vi "Remove_Destination.vi"(6 "defaultDir in":string, 7 "dest tag":string, 8 "error in (no error)":errorcluster, 9 "source in":refnum<class "IB_Source.lvclass">[](array[class]), 10 "destinations in":refnum<class "IB_Destination.lvclass">[](array[class]), 11 "IB_DestTree in":refnum<class "IB_Tree_Dest.lvclass">) -> (0 "error out":errorcluster, 1 "source out":refnum<class "IB_Source.lvclass">[](array[class]), 2 "destinations out":refnum<class "IB_Destination.lvclass">[](array[class]), 3 "IB_DestTree out":refnum<class "IB_Tree_Dest.lvclass">, 4 "defaultDir out":string, 5 "edit":T1)   [LabVIEW 2020, in "IB_Tree_Dest.lvclass"]
uses:
  <vilib>/AppBuilder/IB_Classes/Tree_Dest/IB_Tree_Dest.lvclass
  <vilib>/AppBuilder/IB_Classes/Tree_Dest/IB_Tree_Dest.lvclass/IB_Tree_Dest.ctl
  <vilib>/AppBuilder/IB_Classes/Tree/IB_Tree.lvclass
  <vilib>/AppBuilder/IB_Classes/Destination/IB_Destination.lvclass
  <vilib>/AppBuilder/IB_Classes/Source/IB_Source.lvclass
  <vilib>/AppBuilder/IB_Classes/Tree_Dest/destEdits_operation.ctl
  <vilib>/AppBuilder/IB_Classes/Tree_Dest/destEdits_edit.ctl
  <vilib>/AppBuilder/IB_Classes/Tree_Dest/destEdits_remove.ctl
  e:/builds/penguin/labview/branches/2020/dev/dist/vi.lib/AppBuilder/IB_Classes/Tree/IB_Tree.lvclass
  e:/builds/penguin/labview/branches/2020/dev/dist/vi.lib/AppBuilder/IB_Classes/Tree_Dest/IB_Tree_Dest.lvclass
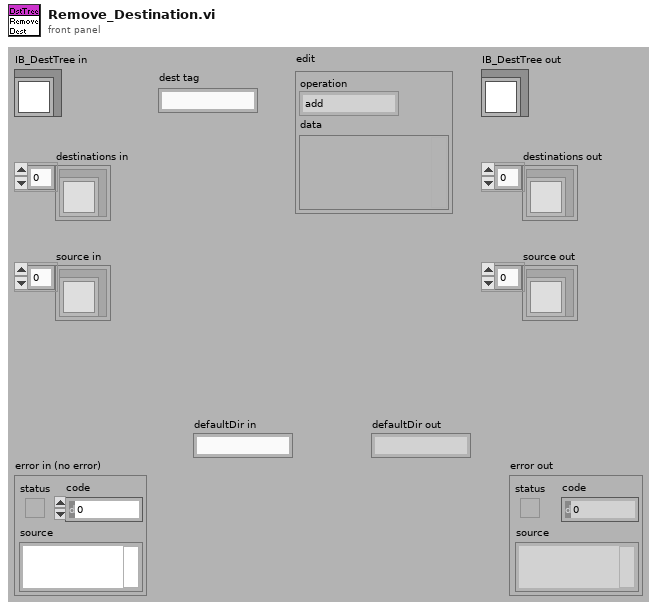
[diagram p1: front panel]
types:
  T1 = typedef "destEdits_edit.ctl" = cluster{"operation":T2, "data":variant}
  T2 = typedef "destEdits_operation.ctl" = enum16{"add", "remove", "rename", "sort children", "default dir changed"}
  T3 = typedef "destEdits_remove.ctl" = cluster{"child tag":string}
  T4 = typedef "IB_Source.ctl" = cluster{"name":string, "sourceTag":string, "destTag":string, "path":path, "eng_installPath":string, "UI_inBuild?":bool, "str ref?":bool}
  T5 = typedef "IB_Destination.ctl" = cluster{"name":string, "unlock":bool, "parentTag":string, "destTag":string, "eng_installPath":string}
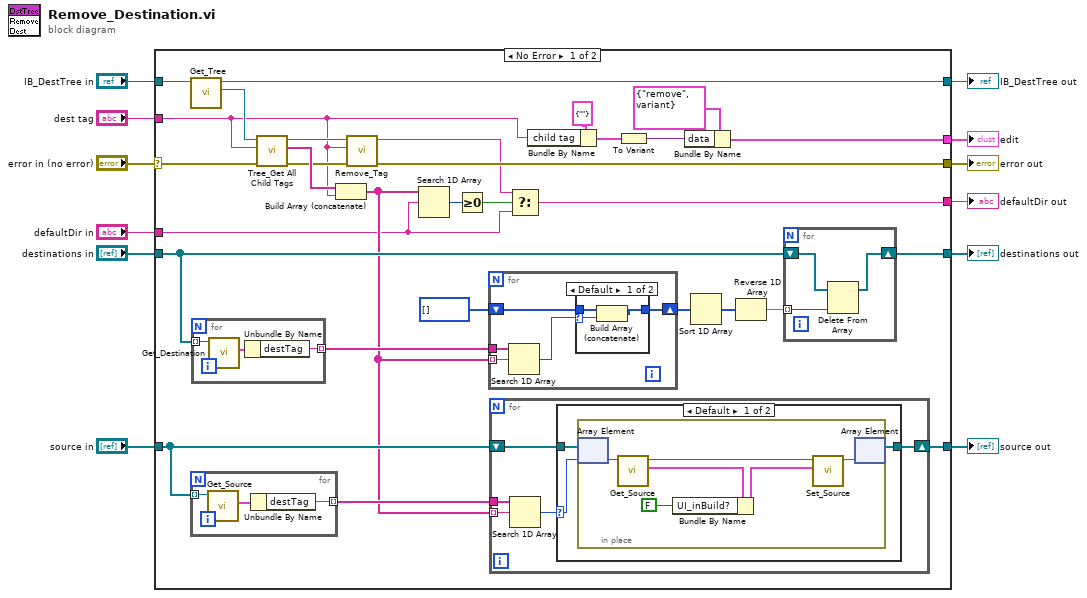
[diagram p0: block diagram]
diagram:
  n1 = case shown="No Error" "error in (no error)" {
    selector: "error in (no error)" -> [w38 w79]
    tunnel: [w29 w79] -> w11
    tunnel: [w40 w78] -> w9
    tunnel: "IB_DestTree in" -> [w41 w78]
    tunnel: "destinations in" -> [w33 w77]
    tunnel: "dest tag" -> [w18 _]
    tunnel: [w22 _] -> w6
    tunnel: [w32 w77] -> w5
    tunnel: "source in" -> [w21 w76]
    tunnel: [w20 w76] -> w3
    tunnel: "defaultDir in" -> [w15 _]
    tunnel: [w17 _] -> w1
    frame No Error {
      n2 = call <vilib>:"Get_Tree.vi"("IB_Tree in"=w41) -> ("ctl"=w42:refnum<vi>, "IB_Tree out"=w40:refnum<class "IB_Tree_Dest.lvclass">)  [unwired: 8 in, 1 out]
      n3 = for {
        tunnel: w21 -> [w60] mode=indexing
        tunnel: [w58] -> w30 mode=indexing
        n4 = call <vilib>:"Get_Source.vi"("IB_Source in"=w60) -> ("data"=w59:T4)  [unwired: 8 in, 2 out]
        n5 = Unbundle By Name(w59) -> ("destTag"=w58:string)
      }
      n6 = for {
        tunnel: w33 -> [w75] mode=indexing
        tunnel: [w73] -> w37 mode=indexing
        n7 = call <vilib>:"Get_Destination.vi"("IB_Destination in"=w75) -> ("data"=w74:T5)  [unwired: 8 in, 2 out]
        n8 = Unbundle By Name(w74) -> ("destTag"=w73:string)
      }
      n9 = call <vilib>:"Tree_Get All Child Tags.vi"("error in (no error)"=w38, "Parent Tag"=w18, "Tree Refnum"=w42) -> ("error out"=w28:errorcluster, "All Child Tags"=w39:string[], "dup Tree Refnum"=w27:refnum<vi>)  [unwired: 6 in]
      n10 = Build Array (concatenate)(w39, w18) -> (w16:string[])
      n11 = call <vilib>:"Remove_Tag.vi"("error in"=w28, "tag"=w18, "Tree Refnum"=w27) -> ("error out"=w29:errorcluster, "selected tag"=w19:string)  [unwired: 7 in]
      n12 = Search 1D Array(1D array=w16, element=w15) -> (index of element=w14:i32)  [unwired: 1 in]
      n13 = Greater Or Equal To 0?(x=w14) -> (x >= 0?=w13:bool)
      n14 = for {
        tunnel: w16 -> [w67] mode=indexing
        tunnel: w37 -> [w68]
        shift-right: [w64] -> w35
        shift-left: i32[] [] -> [w65]
        n15 = Search 1D Array(1D array=w68, element=w67) -> (index of element=w66:i32)  [unwired: 1 in]
        n16 = case shown="Default" w66 {
          selector: w66 -> [w69 _]
          tunnel: w65 -> [w71 w72]
          tunnel: [w70 w72] -> w64
          frame Default {
            n17 = Build Array (concatenate)(w71, w69) -> (w70:i32[])
          }
          frame -1 {
          }
        }
      }
      n18 = for {
        tunnel: w16 -> [w46] mode=indexing
        tunnel: w30 -> [w47]
        shift-right: [w43] -> w20
        shift-left: w21 -> [w44]
        n19 = Search 1D Array(1D array=w47, element=w46) -> (index of element=w45:i32)  [unwired: 1 in]
        n20 = case shown="Default" w45 {
          selector: w45 -> [w49 _]
          tunnel: w44 -> [w50 w57]
          tunnel: [w48 w57] -> w43
          frame Default {
            n21 = in-place {
              n22 = in-place-array #1(w50, w49) -> (w56:refnum<class "IB_Source.lvclass">)
              n23 = call <vilib>:"Get_Source.vi"("IB_Source in"=w56) -> ("data"=w54:T4, "IB_Source out"=w52:refnum<class "IB_Source.lvclass">)  [unwired: 8 in, 1 out]
              n24 = Bundle By Name(cluster=w54, "UI_inBuild?"=FALSE) -> (w53:T4)
              n25 = call <vilib>:"Set_Source.vi"("data"=w53, "IB_Source in"=w52) -> ("IB_Source out"=w55:refnum<class "IB_Source.lvclass">)  [unwired: 8 in, 1 out]
              n26 = in-place-array #1(w55) -> (w48:refnum<class "IB_Source.lvclass">[])  [unwired: 1 out]
            }
          }
          frame -1 {
          }
        }
      }
      n27 = Select(t=w19, s=w13, f=w15) -> (s? t:f=w17:string)
      n28 = Bundle By Name(cluster=T3 {"child tag"=""} ("remove"), "child tag"=w18) -> (w26:T3)
      n29 = To Variant(anything=w26) -> (Variant=w25:variant)
      n30 = Bundle By Name(cluster=T1 {"operation"=enum."remove", "data"=variant} ("edit"), "data"=w25) -> (w22:T1)
      n31 = Sort 1D Array(array=w35) -> (sorted array=w31:i32[])
      n32 = Reverse 1D Array(array=w31) -> (reversed array=w34:i32[])
      n33 = for {
        tunnel: w34 -> [w61] mode=indexing
        shift-right: [w62] -> w32
        shift-left: w33 -> [w63]
        n34 = Delete From Array(array=w63, index=w61) -> (array with subset deleted=w62:refnum<class "IB_Destination.lvclass">[])  [unwired: 1 in, 1 out]
      }
    }
    frame Error {
    }
  }
  "error out" <- w11
  "IB_DestTree out" <- w9
  "destinations out" <- w5
  "edit" <- w6
  "source out" <- w3
  "defaultDir out" <- w1
